vi "MGI Gaussian Smooth.vi"(1 "Accuracy Factor (0.05)":sgl=0.05, 2 "Smooth Columns?":bool, 3 "Smooth Scale":sgl, 4 "Array[][]":sgl[][](array[numeric])) -> (0 "Smoothed Array[][]":sgl[][](array[numeric]))   [LabVIEW 2016]
doc: "Apply a gaussian smoothing function in one direction on a 2D array of data. Smooth scale is the e-fold length in array index units. Accuracy factor is the ratio of the smallest included term to the largest term. Data is effectively surrounded by zero's on the boundary.\n\nAuthored by David A. Moore\nsupport@mooregoodideas.com\nwww.mooregoodideas.com\n\nCopyright (c) 2010, Moore Good Ideas, Inc.\n\nAll rights reserved.\n\nRedistribution and use in source and binary forms, with or without modification, are permitted provided that the following conditions are met:\n\n * Redistributions of source code must retain the above copyright notice, this list of conditions and the following disclaimer.\n * Redistributions in binary form must reproduce the above copyright notice, this list of conditions and the following disclaimer in the documentation and/or other materials provided with the distribution.\n * Neither the name of Moore Good Ideas, Inc. nor the names of its contributors may be used to endorse or promote products derived from this software without specific prior written permission.\n\nTHIS SOFTWARE IS PROVIDED BY THE COPYRIGHT HOLDERS AND CONTRIBUTORS \"AS IS\" AND ANY EXPRESS OR IMPLIED WARRANTIES, INCLUDING, BUT NOT LIMITED TO, THE IMPLIED WARRANTIES OF MERCHANTABILITY AND FITNESS FOR A PARTICULAR PURPOSE ARE DISCLAIMED. IN NO EVENT SHALL THE COPYRIGHT OWNER OR CONTRIBUTORS BE LIABLE FOR ANY DIRECT, INDIRECT, INCIDENTAL, SPECIAL, EXEMPLARY, OR CONSEQUENTIAL DAMAGES (INCLUDING, BUT NOT LIMITED TO, PROCUREMENT OF SUBSTITUTE GOODS OR SERVICES; LOSS OF USE, DATA, OR PROFITS; OR BUSINESS INTERRUPTION) HOWEVER CAUSED AND ON ANY THEORY OF LIABILITY, WHETHER IN CONTRACT, STRICT LIABILITY, OR TORT (INCLUDING NEGLIGENCE OR OTHERWISE) ARISING IN ANY WAY OUT OF THE USE OF THIS SOFTWARE, EVEN IF ADVISED OF THE POSSIBILITY OF SUCH DAMAGE."
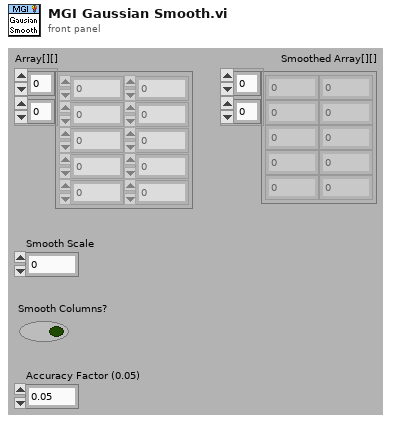
[diagram p1: front panel]
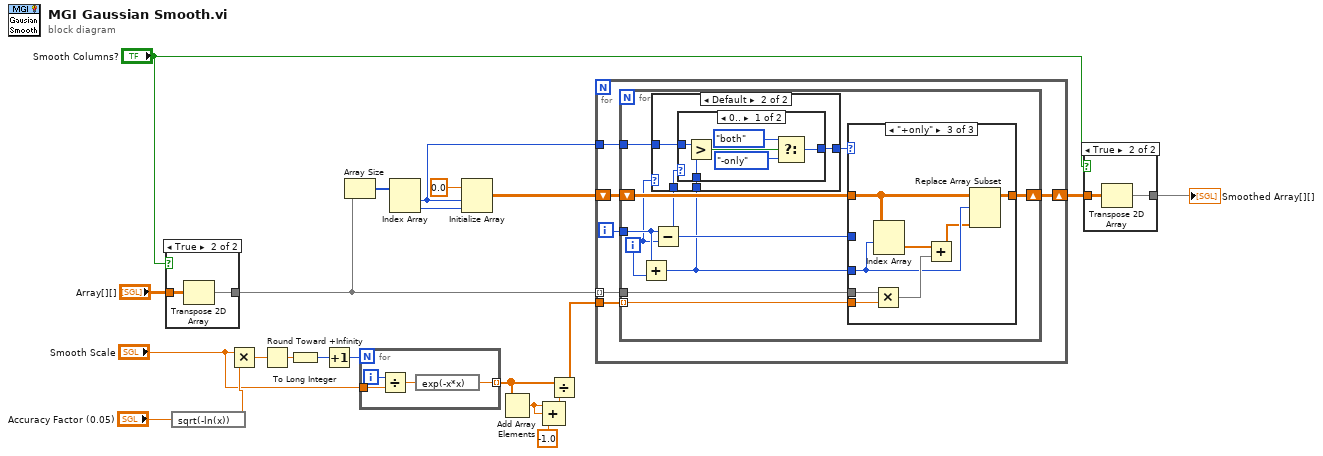
[diagram p0: block diagram]
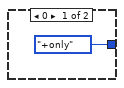
[diagram p3: hidden frame]
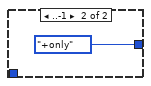
[diagram p4: hidden frame]
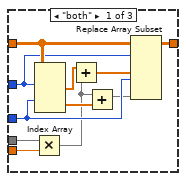
[diagram p5: hidden frame]
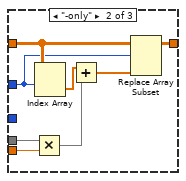
[diagram p6: hidden frame]
diagram:
  n1 = case shown="True" "Smooth Columns?" {
    tunnel: "Array[][]" -> [w23 w25]
    tunnel: [w23 w24] -> w12
    frame False {
    }
    frame True {
      n2 = Transpose 2D Array(2D array=w25) -> (transposed array=w24:sgl[][])
    }
  }
  n3 = expression code="sqrt(-ln(x))"("Accuracy Factor (0.05)") -> (w20:sgl)
  n4 = Multiply(x="Smooth Scale", y=w20) -> (x*y=w19:sgl)
  n5 = Round Toward +Infinity(x=w19) -> (ceil(x): smallest int >= x=w18:sgl)
  n6 = To Long Integer(number=w18) -> (32bit integer=w6:i32)
  n7 = Increment(x=w6) -> (x+1=w7:i32)
  n8 = Array Size(array=w12) -> (size(s)=w11:i32[])
  n9 = for {
    N: w7 -> [_]
    tunnel: "Smooth Scale" -> [w28]
    tunnel: [w26] -> w14 mode=indexing
    i -> [w29]
    n10 = Divide(x=w29, y=w28) -> (x/y=w27:sgl)
    n11 = expression code="exp(-x*x)"(w27) -> (w26:sgl)
  }
  n12 = Index Array(array=w11) -> (element #1=w5:i32, element #2=w10:i32)  [unwired: 2 in]
  n13 = Initialize Array(sgl 0.0, w5, w10) -> (w8:sgl[][])
  n14 = Add Array Elements(numeric array=w14) -> (sum=w16:sgl)
  n15 = Compound Arithmetic op=ADD(w16, w16, sgl -1.0 ("value")) -> (w13:sgl)
  n16 = Divide(x=w14, y=w13) -> (x/y=w4:sgl[])
  n17 = for {
    tunnel: w12 -> [w34] mode=indexing
    shift-right: [w32] -> w3
    shift-left: w8 -> [w35]
    tunnel: w4 -> [w33]
    tunnel: w5 -> [w30]
    i -> [w31]
    n18 = for {
      tunnel: w34 -> [w44]
      tunnel: w33 -> [w43] mode=indexing
      shift-right: [w42] -> w32
      shift-left: w35 -> [w45]
      tunnel: w31 -> [w41]
      tunnel: w30 -> [w37]
      i -> [w40]
      n19 = Add(x=w41, y=w40) -> (x+y=w36:i32)
      n20 = Subtract(x=w41, y=w40) -> (x-y=w38:i32)
      n21 = case shown="Default" w40 {
        tunnel: [enum16{"both", "-only", "+only"}."+only" w49] -> w39
        tunnel: w38 -> [_ w50]
        tunnel: w37 -> [_ w48]
        tunnel: w36 -> [_ w47]
        frame 0 {
        }
        frame Default {
          n22 = case shown="0.." w50 {
            tunnel: [w51 enum16{"both", "-only", "+only"}."+only"] -> w49
            tunnel: w48 -> [w56 _]
            tunnel: w47 -> [w55 _]
            frame 0.. {
              n23 = Greater?(x=w56, y=w55) -> (0:w54:bool)
              n24 = Select(t=enum16{"both", "-only", "+only"}."both", s=w54, f=enum16{"both", "-only", "+only"}."-only") -> (s? t:f=w51:enum16{"both", "-only", "+only"})
            }
            frame ..-1 {
            }
          }
        }
      }
      n25 = case shown="\"+only\"" w39 {
        tunnel: w45 -> [w68 w76 w84]
        tunnel: w44 -> [w67 w75 w83]
        tunnel: w43 -> [w66 w74 w82]
        tunnel: [w65 w73 w81] -> w42
        tunnel: w38 -> [w63 w71 _]
        tunnel: w36 -> [w62 _ w78]
        frame "both" {
          n26 = Multiply(x=w67, y=w66) -> (x*y=w59:sgl[])
          n27 = Index Array(array=w68, index (row) #1=w63, index (row) #2=w62) -> (element #1=w64:sgl[], element #2=w60:sgl[])  [unwired: 2 in]
          n28 = Add(x=w64, y=w59) -> (x+y=w61:sgl[])
          n29 = Add(x=w59, y=w60) -> (x+y=w58:sgl[])
          n30 = Replace Array Subset(array=w68, new element #1=w61, index (row) #1=w63, new element #2=w58, index (row) #2=w62) -> (w65:sgl[][])  [unwired: 2 in]
        }
        frame "-only" {
          n31 = Multiply(x=w75, y=w74) -> (x*y=w69:sgl[])
          n32 = Index Array(array=w76, index (row)=w71) -> (element=w72:sgl[])  [unwired: 1 in]
          n33 = Add(x=w72, y=w69) -> (x+y=w70:sgl[])
          n34 = Replace Array Subset(array=w76, new element=w70, index (row)=w71) -> (w73:sgl[][])  [unwired: 1 in]
        }
        frame "+only" {
          n35 = Multiply(x=w83, y=w82) -> (x*y=w79:sgl[])
          n36 = Index Array(array=w84, index (row)=w78) -> (element=w80:sgl[])  [unwired: 1 in]
          n37 = Add(x=w80, y=w79) -> (x+y=w77:sgl[])
          n38 = Replace Array Subset(array=w84, new element=w77, index (row)=w78) -> (w81:sgl[][])  [unwired: 1 in]
        }
      }
    }
  }
  n39 = case shown="True" "Smooth Columns?" {
    tunnel: w3 -> [w85 w87]
    tunnel: [w85 w86] -> w2
    frame False {
    }
    frame True {
      n40 = Transpose 2D Array(2D array=w87) -> (transposed array=w86:sgl[][])
    }
  }
  "Smoothed Array[][]" <- w2
